vi "open_visa_resources.vi"(8 "error in (no error)":errorcluster, 10 "test mode":T1(ring), 11 "config file in":string="VISA_config.ini") -> (0 "error out":errorcluster, 3 "VISA out":T2)   [LabVIEW 2015]
uses:
  Type Definitions/get_visa_resources_states.ctl
  Type Definitions/get_visa_resources_data.ctl
panel:
  # "There are four possible test modes:\ntest_mode = 0 : Hi-Pot--->GB\ntest_mode = 1 : GB--->Hi-Pot\ntest_mode = 2 : Hi-Pot only (Default)\ntest_mode = 3 : GB only"
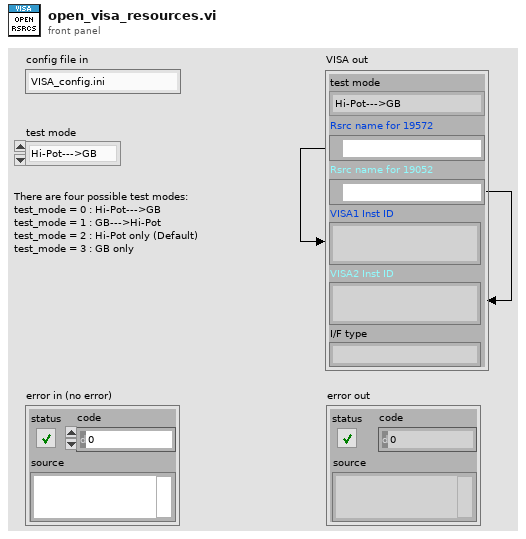
[diagram p1: front panel]
types:
  T1 = enum16{"Hi-Pot--->GB", "GB--->Hi-Pot", "Hi-Pot only", "GB only"}
  T2 = cluster{"Rsrc name for 19572":refnum<visa-resource-name>, "Rsrc name for 19052":refnum<visa-resource-name>, "I/F type":string, "VISA2 Inst ID":string, "VISA1 Inst ID":string, "test mode":enum16{"Hi-Pot--->GB", "GB--->Hi-Pot", "Hi-Pot only", "GB only"}}
  T3 = typedef "get_visa_resources_data.ctl" = cluster{"19052 COM":cluster{"COM port":string, "b rate":string, "f control":string, "parity":string}, "19572 COM":cluster{"COM port":string, "b rate":string, "f control":string, "parity":string}, "Assgs":cluster{"VISA1 Inst ID":string, "VISA2 Inst ID":string, "I/F type":string}, "test mode":enum16{"Hi-Pot--->GB", "GB--->Hi-Pot", "Hi-Pot only", "GB only"}}
  T4 = typedef "get_visa_resources_states.ctl" = enum16{"Initialize", "Get Interface type", "Build VISA Rsrc Name (GPIB)", "Build VISA Rsrc Name (RS232)", "Set RS232 parameters", "Get Instrument ID(s)", "Shutdown"}
  T5 = cluster{"gpib_board_No.":string, "19572_gpib_prim_adr":string, "19052_gpib_prim_adr":string}
  T6 = cluster{"COM port":string, "baud rate":string, "flow control":string, "parity":string}
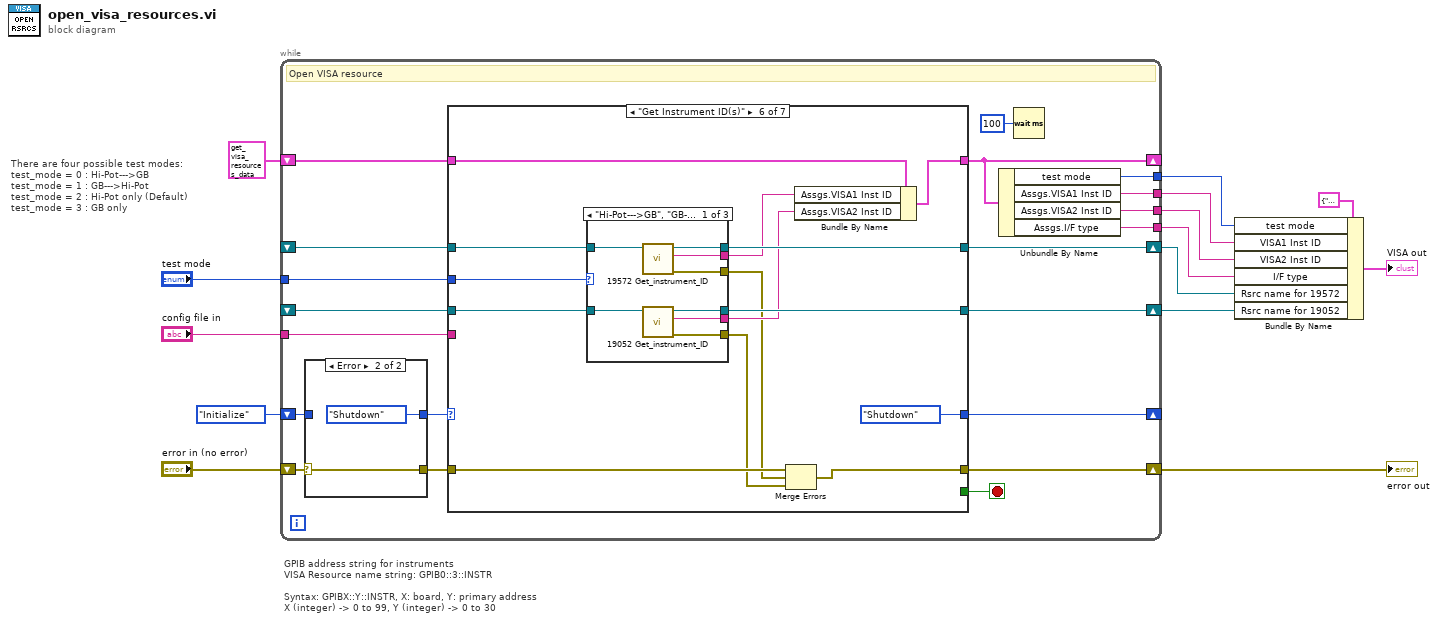
[diagram p0: block diagram]
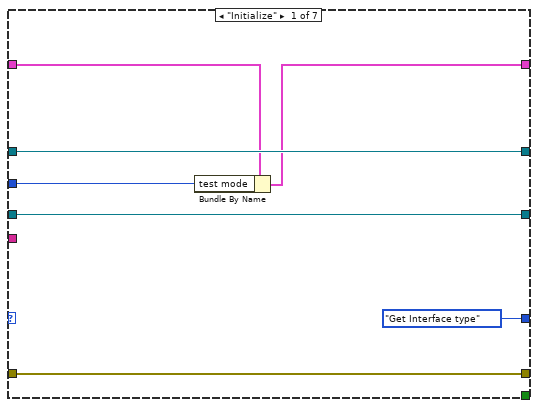
[diagram p3: hidden frame]
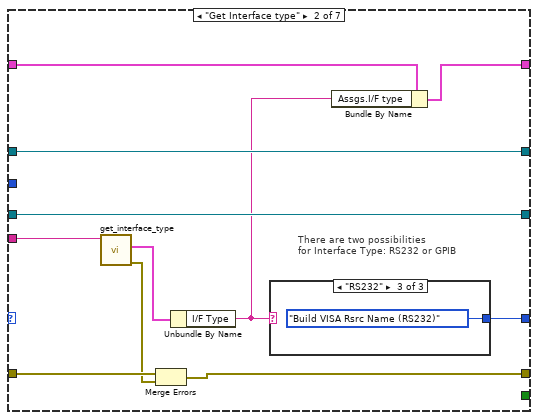
[diagram p4: hidden frame]
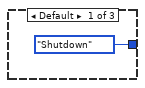
[diagram p5: hidden frame]
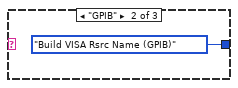
[diagram p6: hidden frame]
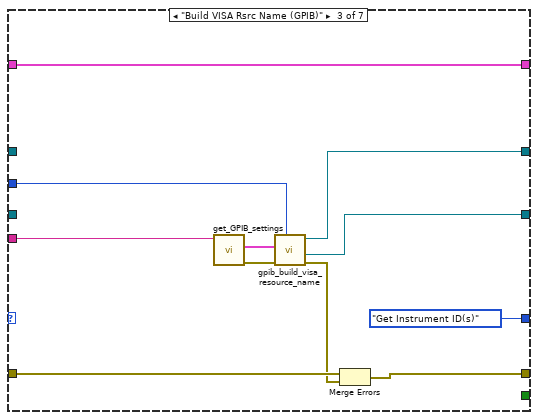
[diagram p7: hidden frame]
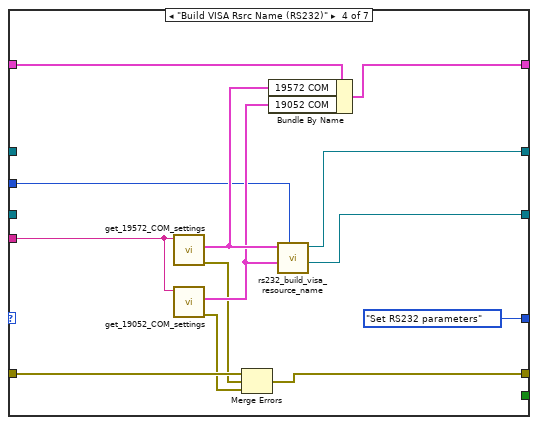
[diagram p8: hidden frame]
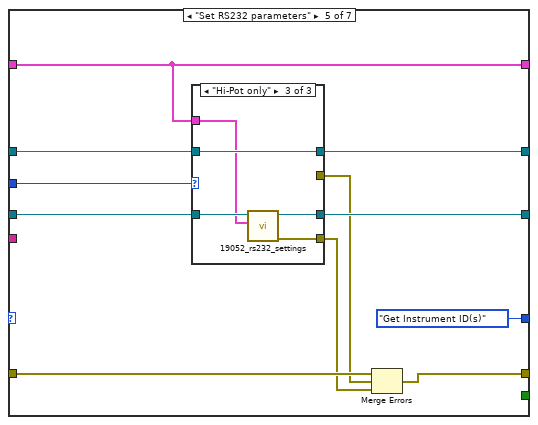
[diagram p9: hidden frame]
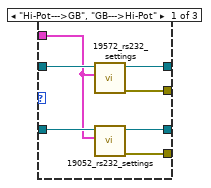
[diagram p10: hidden frame]
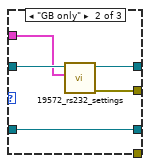
[diagram p11: hidden frame]
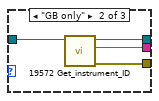
[diagram p12: hidden frame]
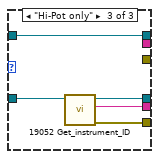
[diagram p13: hidden frame]
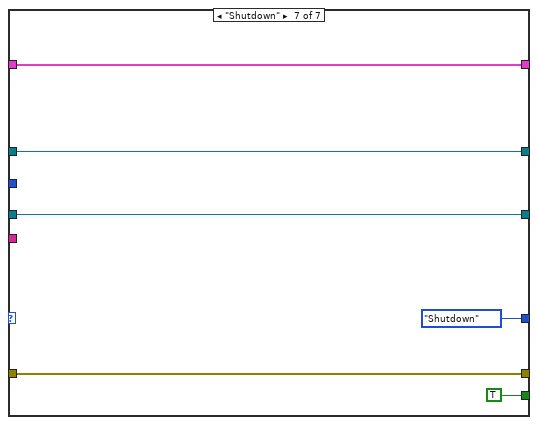
[diagram p14: hidden frame]
diagram:
  # "There are four possible test modes:\ntest_mode = 0 : Hi-Pot--->GB\ntest_mode = 1 : GB--->Hi-Pot\ntest_mode = 2 : Hi-Pot only (Default)\ntest_mode = 3 : GB only"
  # "GPIB address string for instruments\nVISA Resource name string: GPIB0::3::INSTR\n\nSyntax: GPIBX::Y::INSTR, X: board, Y: primary address\nX (integer) -> 0 to 99, Y (integer) -> 0 to 30"
  n1 = while {
    shift-right: [w32] -> w13
    shift-left: "error in (no error)" -> [w34]
    shift-right: [w29] -> _
    shift-left: get_visa_resources_states."Initialize" -> [w31]
    tunnel: "test mode" -> [w27]
    shift-right: [w24] -> _
    shift-left: T3 {"19052 COM"={"COM port"="", "b rate"="", "f control"="", "parity"=""}, "19572 COM"={"COM port"="", "b rate"="", "f control"="", "parity"=""}, "Assgs"={"VISA1 Inst ID"="", "VISA2 Inst ID"="", "I/F type"=""}, "test mode"=enum."Hi-Pot--->GB"} -> [w26]
    tunnel: "config file in" -> [w25]
    tunnel: [w22] -> w7
    shift-right: [w21] -> w9
    shift-left: _ -> [w19]
    shift-right: [w20] -> w8
    shift-left: _ -> [w18]
    tunnel: [w17] -> w6
    tunnel: [w16] -> w5
    tunnel: [w15] -> w1
    stop <- w28 stop-if-true
    # "Open VISA resource"
    n2 = case shown="Error" w34 {
      selector: w34 -> [w36 w38]
      tunnel: [w36 w38] -> w33
      tunnel: w31 -> [w35 _]
      tunnel: [w35 get_visa_resources_states."Shutdown"] -> w30
      frame No Error {
      }
      frame Error {
      }
    }
    n3 = case shown="\"Get Instrument ID(s)\"" w30 {
      tunnel: w33 -> [w45 w47 w61 w73 w86 w114 w148]
      tunnel: [w45 w48 w62 w75 w93 w117 w148] -> w32
      tunnel: [get_visa_resources_states."Get Interface type" w55 get_visa_resources_states."Get Instrument ID(s)" get_visa_resources_states."Set RS232 parameters" get_visa_resources_states."Get Instrument ID(s)" get_visa_resources_states."Shutdown" get_visa_resources_states."Shutdown"] -> w29
      tunnel: [_ _ _ _ _ _ TRUE] -> w28
      tunnel: w27 -> [w39 _ w67 w74 w94 w125 _]
      tunnel: w26 -> [w41 w54 w65 w82 w88 w115 w147]
      tunnel: [w40 w53 w65 w81 w88 w124 w147] -> w24
      tunnel: w25 -> [_ w56 w70 w79 _ _ _]
      tunnel: [w43 w52 w66 w80 w91 w120 w144] -> w21
      tunnel: [w42 w51 w64 w77 w89 w119 w143] -> w20
      tunnel: w19 -> [w43 w52 _ _ w92 w122 w144]
      tunnel: w18 -> [w42 w51 _ _ w90 w121 w143]
      frame "Initialize" {
        n4 = Bundle By Name(cluster=w41, "test mode"=w39) -> (w40:T3)
      }
      frame "Get Interface type" {
        # "There are two possibilities\nfor Interface Type: RS232 or GPIB"
        n5 = call "get_interface_type.vi"("config_file_name"=w56) -> ("error out"=w46:errorcluster, "Data"=w50:cluster{"I/F Type":string})  [unwired: 8 in, 1 out]
        n6 = Merge Errors(w47, w46) -> (w48:errorcluster)
        n7 = Unbundle By Name(w50) -> ("I/F Type"=w49:string)
        n8 = case shown="\"RS232\"" w49 {
          tunnel: [get_visa_resources_states."Shutdown" get_visa_resources_states."Build VISA Rsrc Name (GPIB)" get_visa_resources_states."Build VISA Rsrc Name (RS232)"] -> w55
          frame Default {
          }
          frame "GPIB" {
          }
          frame "RS232" {
          }
        }
        n9 = Bundle By Name(cluster=w54, "Assgs.I/F type"=w49) -> (w53:T3)
      }
      frame "Build VISA Rsrc Name (GPIB)" {
        n10 = call "get_GPIB_settings.vi"("config_file_name"=w70) -> ("error out"=w69:errorcluster, "GPIB settings"=w68:T5)  [unwired: 8 in, 1 out]
        n11 = call "gpib_build_visa_resource_name.vi"("test mode"=w67, "error in (no error)"=w69, "GPIB settings"=w68) -> ("error out"=w60:errorcluster, "VISA Resource name 2"=w64:refnum<visa-resource-name>, "VISA Resource name 1"=w66:refnum<visa-resource-name>)  [unwired: 6 in]
        n12 = Merge Errors(w61, w60) -> (w62:errorcluster)
      }
      frame "Build VISA Rsrc Name (RS232)" {
        n13 = call "get_19572_COM_settings.vi"("config_file_name"=w79) -> ("error out"=w71:errorcluster, "19572 COM settings"=w83:T6)  [unwired: 8 in, 1 out]
        n14 = call "get_19052_COM_settings.vi"("config_file_name"=w79) -> ("error out"=w72:errorcluster, "19052 COM settings"=w78:T6)  [unwired: 8 in, 1 out]
        n15 = Merge Errors(w73, w71, w72) -> (w75:errorcluster)
        n16 = Bundle By Name(cluster=w82, "19572 COM"=w83, "19052 COM"=w78) -> (w81:T3)
        n17 = call "rs232_build_visa_resource_name.vi"("test mode"=w74, "19052 COM settings"=w78, "19572 COM settings"=w83) -> ("VISA Resource name 2"=w77:refnum<visa-resource-name>, "VISA Resource name 1"=w80:refnum<visa-resource-name>)  [unwired: 7 in]
      }
      frame "Set RS232 parameters" {
        n18 = case shown="\"Hi-Pot only\"" w94 {
          tunnel: [w101 w106 _] -> w84
          tunnel: w88 -> [w95 w103 w107]
          tunnel: [w100 _ w111] -> w85
          tunnel: w92 -> [w97 w104 w110]
          tunnel: [w99 w105 w110] -> w91
          tunnel: w90 -> [w96 w102 w108]
          tunnel: [w98 w102 w109] -> w89
          frame "Hi-Pot--->GB", "GB--->Hi-Pot" {
            n19 = call "19572_rs232_settings.vi"("input cluster"=w95, "reference in"=w97) -> ("error out"=w101:errorcluster, "reference out"=w99:refnum<visa-resource-name>)  [unwired: 8 in]
            n20 = call "19052_rs232_settings.vi"("input cluster"=w95, "reference in"=w96) -> ("error out"=w100:errorcluster, "reference out"=w98:refnum<visa-resource-name>)  [unwired: 8 in]
          }
          frame "GB only" {
            n21 = call "19572_rs232_settings.vi"("input cluster"=w103, "reference in"=w104) -> ("error out"=w106:errorcluster, "reference out"=w105:refnum<visa-resource-name>)  [unwired: 8 in]
          }
          frame "Hi-Pot only" {
            n22 = call "19052_rs232_settings.vi"("input cluster"=w107, "reference in"=w108) -> ("error out"=w111:errorcluster, "reference out"=w109:refnum<visa-resource-name>)  [unwired: 8 in]
          }
        }
        n23 = Merge Errors(w86, w84, w85) -> (w93:errorcluster)
      }
      frame "Get Instrument ID(s)" {
        n24 = case shown="\"Hi-Pot--->GB\", \"GB--->Hi-Pot\"" w125 {
          tunnel: w122 -> [w133 w137 w139]
          tunnel: w121 -> [w131 _ w142]
          tunnel: [w132 w136 _] -> w118
          tunnel: [w128 _ w141] -> w116
          tunnel: [w130 w135 w139] -> w120
          tunnel: [w129 _ w140] -> w119
          tunnel: [w127 w134 _] -> w112
          tunnel: [w126 _ w138] -> w113
          frame "Hi-Pot--->GB", "GB--->Hi-Pot" {
            n25 = call "19572 Get_instrument_ID.vi"("VISA resource name in"=w133) -> ("error out"=w127:errorcluster, "instrument ID"=w132:string, "VISA resource name out"=w130:refnum<visa-resource-name>)  [unwired: 8 in]
            n26 = call "19052 Get_instrument_ID.vi"("VISA resource name in"=w131) -> ("error out"=w126:errorcluster, "instrument ID"=w128:string, "VISA resource name out"=w129:refnum<visa-resource-name>)  [unwired: 8 in]
          }
          frame "GB only" {
            n27 = call "19572 Get_instrument_ID.vi"("VISA resource name in"=w137) -> ("error out"=w134:errorcluster, "instrument ID"=w136:string, "VISA resource name out"=w135:refnum<visa-resource-name>)  [unwired: 8 in]
          }
          frame "Hi-Pot only" {
            n28 = call "19052 Get_instrument_ID.vi"("VISA resource name in"=w142) -> ("error out"=w138:errorcluster, "instrument ID"=w141:string, "VISA resource name out"=w140:refnum<visa-resource-name>)  [unwired: 8 in]
          }
        }
        n29 = Merge Errors(w114, w112, w113) -> (w117:errorcluster)
        n30 = Bundle By Name(cluster=w115, "Assgs.VISA1 Inst ID"=w118, "Assgs.VISA2 Inst ID"=w116) -> (w124:T3)
      }
      frame "Shutdown" {
      }
    }
    n31 = Unbundle By Name(w24) -> ("test mode"=w15:T1, "Assgs.VISA1 Inst ID"=w22:string, "Assgs.VISA2 Inst ID"=w17:string, "Assgs.I/F type"=w16:string)
    n32 = Wait (ms)(milliseconds to wait=u32 100) -> ()  [unwired: 1 out]
  }
  "error out" <- w13
  n33 = Bundle By Name(cluster=T2 {"Rsrc name for 19572"="", "Rsrc name for 19052"="", "I/F type"="", "VISA2 Inst ID"="", "VISA1 Inst ID"="", "test mode"=enum."Hi-Pot only"} ("VISA out"), "test mode"=w1, "VISA1 Inst ID"=w7, "VISA2 Inst ID"=w6, "I/F type"=w5, "Rsrc name for 19572"=w9, "Rsrc name for 19052"=w8) -> (→"VISA out":T2)
